vi "Unpack Linear Address (SubVI).vi"(11 "Linear Address":u32) -> (0 "Bit Address":u8, 3 "Packet Address":u32)   [LabVIEW 2015]
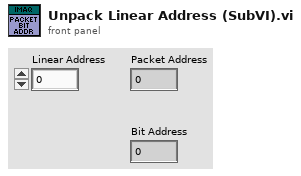
[diagram p1: front panel]
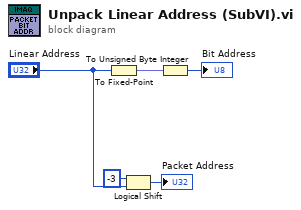
[diagram p0: block diagram]
diagram:
  n1 = To Fixed-Point(number="Linear Address") -> (fixed-point=w1:fxp<+,3,3>)  [unwired: 1 in]
  n2 = Logical Shift(y=i16 -3, x="Linear Address") -> (x << y=→"Packet Address":u32)
  n3 = To Unsigned Byte Integer(number=w1) -> (unsigned 8bit integer=→"Bit Address":u8)
